vi "Both Encoders Control.vi"(0 "Reset Both":bool) -> (1 "Distance Avg (in)":dbl, 2 "Rate Avg":dbl)   [LabVIEW 2013]
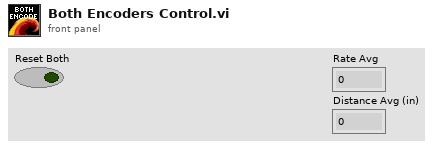
[diagram p1: front panel]
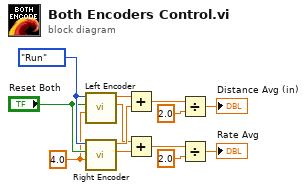
[diagram p0: block diagram]
diagram:
  w11 = 4.0 ("Wheel Size")
  w13 = enum16{"Start", "Run", "End"}."Run" ("Enum")
  n1 = call "Left Encoder.vi"("Wheel Size"=w11, "Reset"="Reset Both", "Enum"=w13) -> ("Rate"=w3:dbl, "Distance (in)"=w10:dbl)  [unwired: 7 in]
  n2 = call "Right Encoder.vi"("Wheel Size"=w11, "Reset"="Reset Both", "Enum"=w13) -> ("Rate"=w4:dbl, "Distance (in)"=w9:dbl)  [unwired: 7 in]
  n3 = Add(x=w10, y=w9) -> (x+y=w8:dbl)
  n4 = Add(x=w3, y=w4) -> (x+y=w5:dbl)
  n5 = Divide(x=w8, y=2.0) -> (x/y=→"Distance Avg (in)":dbl)
  n6 = Divide(x=w5, y=2.0) -> (x/y=→"Rate Avg":dbl)
